vi "VISA_WRITE_2.vi"(5 "Value":i32, 6 "No Value (T)":bool, 7 "Value (str)":string, 8 "error in":errorcluster {"code" format="%.0x"}, 10 "cmd":string, 11 "Session In":refnum<visa-resource-name>="GPIB0::10::INSTR") -> (0 "error out":errorcluster {"code" format="%.0x"}, 2 "concatenated string":string, 3 "Session Out":refnum<visa-resource-name>)   [LabVIEW 2018]
panel:
  # "Use for debugging if no values are entered"
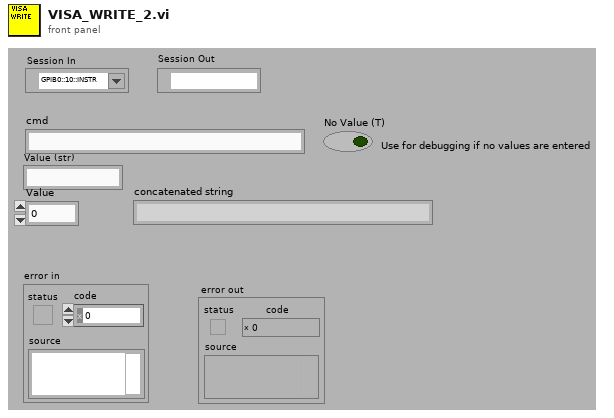
[diagram p1: front panel]
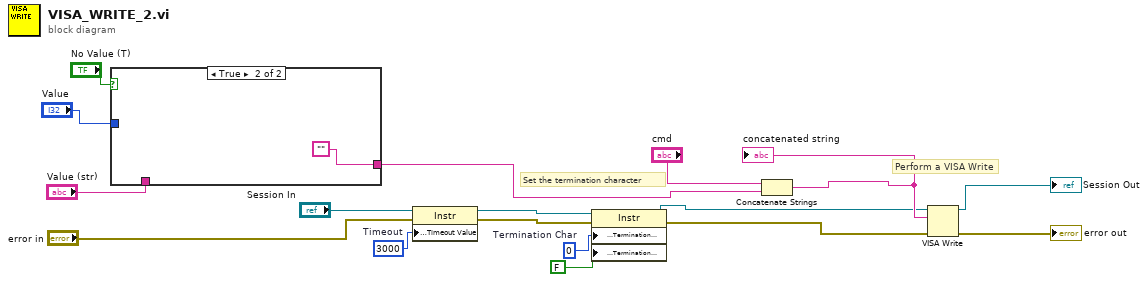
[diagram p0: block diagram]
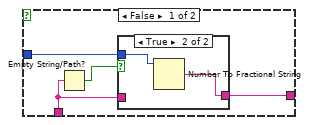
[diagram p2: hidden frame]
diagram:
  w12 = u8 0  # Termination Char
  w16 = u32 3000  # Timeout
  # "Perform a VISA Write"
  # "Set the termination character"
  n1 = case shown="True" "No Value (T)" {
    tunnel: "Value (str)" -> [w21 _]
    tunnel: [w19 ""] -> w3
    tunnel: "Value" -> [w18 _]
    frame False {
      n2 = Empty String/Path?(string/path=w21) -> (empty?=w20:bool)
      n3 = case shown="True" w20 {
        tunnel: w21 -> [w22 _]
        tunnel: [w22 w24] -> w19
        tunnel: w18 -> [_ w23]
        frame False {
        }
        frame True {
          n4 = Number To Fractional String(number=w23) -> (F-format string=w24:string)  [unwired: 3 in]
        }
      }
    }
    frame True {
    }
  }
  n5 = property class="Instr"(reference="Session In", error in="error in", "General Settings:Timeout Value"=w16) -> (reference out=w11:refnum<visa-resource-name>, error out=w14:errorcluster)
  n6 = property class="Instr"(reference=w11, error in=w14, "Message Based Settings:Termination Character"=w12, "Message Based Settings:Termination Character Enable"=FALSE ("enable")) -> (reference out=w6:refnum<visa-resource-name>, error out=w13:errorcluster)
  n7 = Concatenate Strings("cmd", w3) -> (w7:string)
  "concatenated string" <- w7
  n8 = VISA Write(VISA resource name=w6, write buffer=w7, error in (no error)=w13) -> (VISA resource name out=→"Session Out":refnum<visa-resource-name>, error out=→"error out":errorcluster)  [unwired: 1 out]
